vi "Open Driver.vi"(8 "error in (no error)":errorcluster) -> (0 "error out":errorcluster)   [LabVIEW 2015, in "TPVG_DLL.lvlib"]
doc: "Use to create a link between the DLL interface and the\nKernel mode driver\n\n--------------------------------------------------------------\nWritten by: Dang Lam"
uses:
  TPVG_DLL.lvlib
  TPVG_DLL.dll
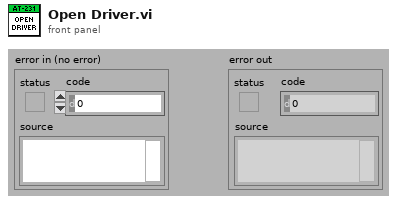
[diagram p1: front panel]
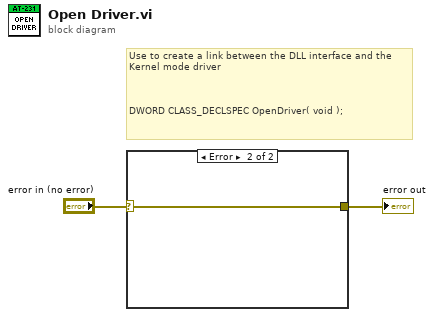
[diagram p0: block diagram]
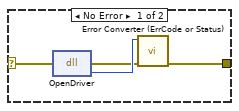
[diagram p2: hidden frame]
diagram:
  # "Use to create a link between the DLL interface and the\nKernel mode driver\n\n\n\nDWORD CLASS_DECLSPEC OpenDriver( void );"
  n1 = case shown="Error" "error in (no error)" {
    selector: "error in (no error)" -> [w3 w7]
    tunnel: [w4 w7] -> w2
    frame No Error {
      n2 = dll-call lib="\\\\Mac\\Home/Desktop/imt_test_app 28-06-2012/TPVG_DLL.dll" fn="OpenDriver"(error in=w3) -> (error out=w5:errorcluster, "return type"=w6:u32)  [unwired: 2 in, 1 out]
      n3 = call "Error Converter (ErrCode or Status).vi"("error in (no error)"=w5, "error code"=w6) -> ("error out"=w4:errorcluster)  [unwired: 9 in]
    }
    frame Error {
    }
  }
  "error out" <- w2
